vi "Harmonics.vi"() -> ()   [LabVIEW 2018]
doc: "PNA-X Example."
uses:
  Instance           1 17Saved   Harmonics .vi
  PNA-X.lvlib
panel:
  out "XY Graph":cluster{dbl[], "Data":dbl[]}(graph)
  out "error out":errorcluster
  out "VISA Out":refnum<visa-resource-name>
  in  "error in":errorcluster
  in  "VISA IN":refnum<visa-resource-name>
  # "1. Select Instrument Source from the \"VISA IN\" drop down.\n2. Run vi"
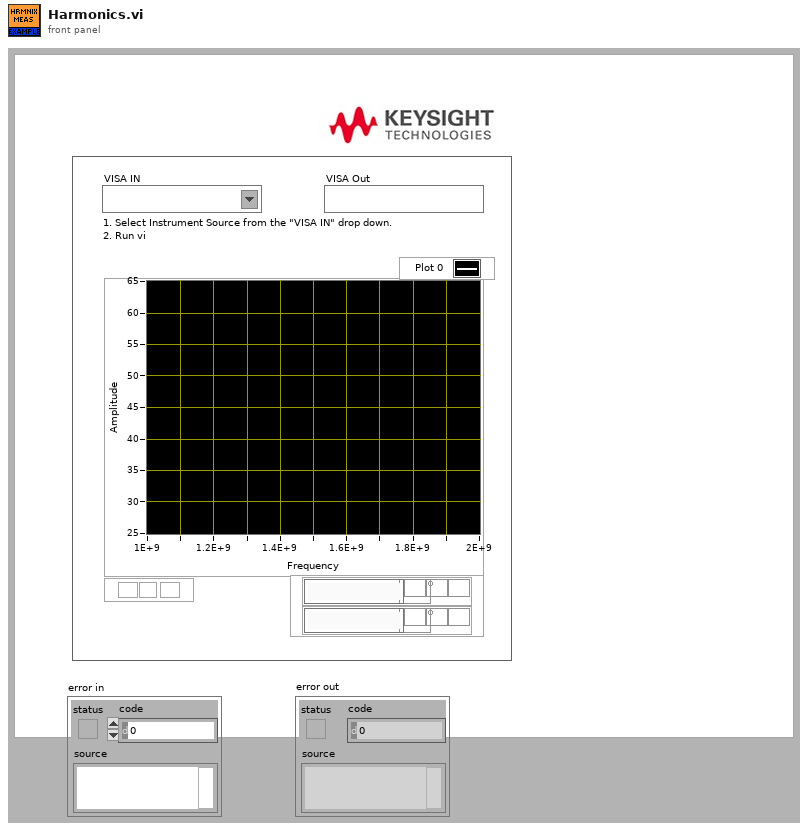
[diagram p1: front panel]
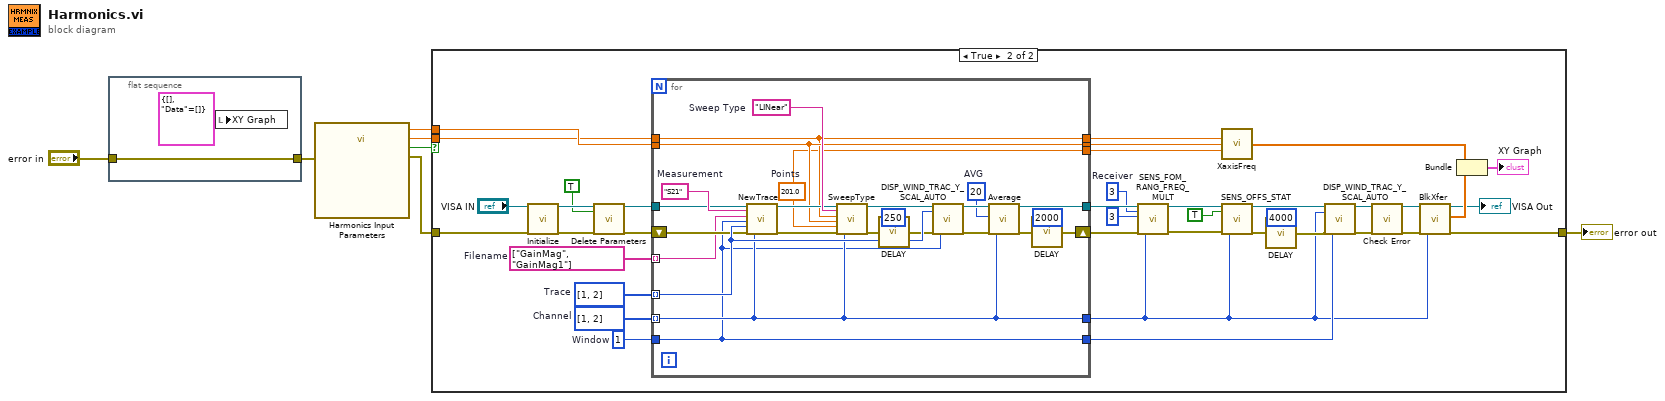
[diagram p0: block diagram]
diagram:
  n1 = flat-sequence {
    tunnel: "error in" -> [w8]
    tunnel: [w8] -> w1
    frame #0 {
      n2 = local write "XY Graph"(cluster{dbl[], "Data":dbl[]} {[], "Data"=[]} ("XY Graph")) -> ()
    }
  }
  n3 = call "Harmonics Input Parameters"("error in (no error)"=w1) -> ("Stop Frequency"=w6:dbl, "Start Frequency"=w5:dbl, "Execute"=w4:bool, "error out"=w3:errorcluster)  [unwired: 15 in]
  n4 = case shown="True" w4 {
    tunnel: [w10 w16] -> w7
    tunnel: w6 -> [_ w24]
    tunnel: w5 -> [_ w23]
    tunnel: w3 -> [w10 w22]
    frame False {
    }
    frame True {
      w42 = string[] ["GainMag", "GainMag1"]  # Filename
      w36 = i32[] [1, 2]  # Channel
      w43 = i32[] [1, 2]  # Trace
      w31 = 1  # Window
      w40 = 3  # Receiver
      n5 = call "Initialize.vi"("VISA IN"="VISA IN", "error in"=w22) -> ("VISA Out"=w48:refnum<visa-resource-name>, "error out"=w46:errorcluster)  [unwired: 15 in, 1 out]
      n6 = call "Delete Parameters .vi"("VISA IN"=w48, "Delete All?"=TRUE, "error in"=w46) -> ("VISA Out"=w44:refnum<visa-resource-name>, "error out"=w45:errorcluster)  [unwired: 15 in]
      n7 = for {
        tunnel: w44 -> [w68]
        tunnel: w43 -> [w71] mode=indexing
        tunnel: w42 -> [w63] mode=indexing
        tunnel: [w60] -> w41
        tunnel: w36 -> [w64] mode=indexing
        tunnel: [w62] -> w35
        shift-right: [w53] -> w27
        shift-left: w45 -> [w69]
        tunnel: [w64] -> w19
        tunnel: w31 -> [w62]
        tunnel: w24 -> [w51]
        tunnel: w23 -> [w50]
        tunnel: [w51] -> w14
        tunnel: [w50] -> w15
        tunnel: [w49] -> w13
        w61 = 20  # AVG
        w49 = 201.0  # Points
        w67 = "LINear"  # Sweep Type
        w72 = "S21"  # Measurement
        n8 = call "NewTrace.vi"("VISA IN"=w68, "Measurement"=w72, "FileName"=w63, "Window"=w62, "Trace"=w71, "error in (no error)"=w69, "Channel"=w64) -> ("VISA Out"=w66:refnum<visa-resource-name>, "error out"=w58:errorcluster)  [unwired: 11 in]
        n9 = call "SweepType.vi"("VISA IN"=w66, "Sweep Type"=w67, "Start Frq."=w50, "Stop Frq."=w51, "Points"=w49, "error in"=w58, "Channel"=w64) -> ("VISA Out"=w65:refnum<visa-resource-name>, "error out"=w57:errorcluster)  [unwired: 11 in]
        n10 = call "DELAY.vi"("milliseconds to wait"=u32 250, "error in (no error)"=w57) -> ("error out"=w56:errorcluster)  [unwired: 13 in]
        n11 = call "DISP_WIND_TRAC_Y_SCAL_AUTO.vi"("VISA IN"=w65, "Trace"=w71, "error in"=w56, "Window"=w62) -> ("VISA Out"=w70:refnum<visa-resource-name>, "error out"=w59:errorcluster)  [unwired: 14 in]
        n12 = call "Average.vi"("VISA IN"=w70, "AVG"=w61, "error in"=w59, "Channel"=w64) -> ("VISA Out"=w60:refnum<visa-resource-name>, "error out"=w54:errorcluster)  [unwired: 14 in]
        n13 = call "DELAY.vi"("milliseconds to wait"=u32 2000, "error in (no error)"=w54) -> ("error out"=w53:errorcluster)  [unwired: 13 in]
      }
      n14 = call "SENS_FOM_RANG_FREQ_MULT.vi"("VISA IN"=w41, "Range number"=w40, "Multiplier Value"=3, "error in"=w27, "Channel"=w19) -> ("VISA Out"=w38:refnum<visa-resource-name>, "error out"=w26:errorcluster)  [unwired: 13 in]
      n15 = call "XaxisFreq.vi"("Start Frequency"=w15, "Stop Frequency"=w14, "Points"=w13) -> ("X-Axis"=w12:dbl[])  [unwired: 12 in]
      n16 = call "SENS_OFFS_STAT.vi"("VISA IN"=w38, "Frq. Offset ON/OFF"=TRUE, "error in"=w26, "Channel"=w19) -> ("VISA Out"=w32:refnum<visa-resource-name>, "error out"=w30:errorcluster)  [unwired: 14 in]
      n17 = call "DELAY.vi"("milliseconds to wait"=u32 4000, "error in (no error)"=w30) -> ("error out"=w29:errorcluster)  [unwired: 13 in]
      n18 = call "DISP_WIND_TRAC_Y_SCAL_AUTO.vi"("VISA IN"=w32, "Trace"=w19, "error in"=w29, "Window"=w35) -> ("VISA Out"=w34:refnum<visa-resource-name>, "error out"=w33:errorcluster)  [unwired: 14 in]
      n19 = call "Check Error.vi"("VISA Resource Name"=w34, "error in (no error)"=w33) -> ("dup VISA session"=w21:refnum<visa-resource-name>, "error out"=w20:errorcluster)  [unwired: 16 in]
      n20 = call "BlkXfer.vi"("VISA IN"=w21, "error in"=w20, "Channel"=w19) -> ("VISA Out"=→"VISA Out":refnum<visa-resource-name>, "Data"=w18:dbl[], "error out"=w16:errorcluster)  [unwired: 14 in]
      n21 = Bundle("X-Axis"=w12, "Data"=w18) -> (→"XY Graph":cluster{"X-Axis":dbl[], "Data":dbl[]})  [unwired: 1 in]
    }
  }
  "error out" <- w7
